vi "Get MAV ID.vi"(8 "Error In":errorcluster, 11 "Aircraft Index":u8) -> (0 "Error Out":errorcluster, 3 "Aircraft ID":u8)   [LabVIEW 2014]
uses:
  Get Aircraft Information.vi
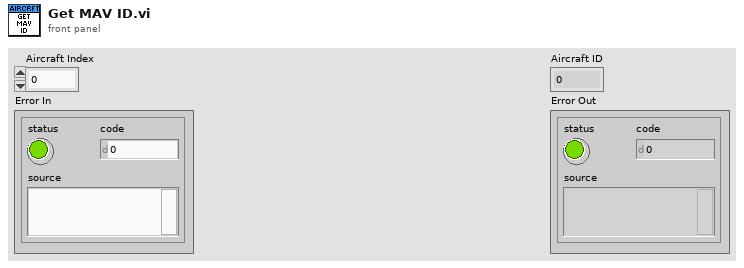
[diagram p1: front panel]
types:
  T1 = typedef "Drone Information.ctl" = cluster{"Aircraft ID":u8, "Tag ID":string, "System Status":string, "Base Mode":T2, "Armed/Disarmed":bool, "Battery Voltage":dbl, "Control Mode":T3, "Initialisation":u8, "Coms with aircraft good":bool, "Mode":string, "Mission Uploaded":bool}
  T2 = typedef "Base Mode.ctl" = cluster{"Custom Mode":bool, "Test Enabled":bool, "Autonomous Mode":bool, "Guided Mode":bool, "Stabilization Enabled":bool, "HIL Enabled":bool, "Manual Mode":bool, "Arm":bool}
  T3 = typedef "Aircraft Mode.ctl" = enum16{"Loiter", "Stabalise", "Failsafe", "Emergency Stop"}
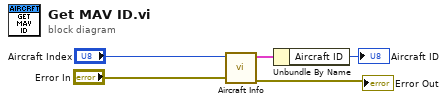
[diagram p0: block diagram]
diagram:
  n1 = call-poly "Aircraft Info.vi"("Error In"="Error In", "Aircraft ID"="Aircraft Index") -> ("Error Out"=→"Error Out":errorcluster, "Aircraft Information Out"=w4:T1)  [unwired: 8 in]
  n2 = Unbundle By Name(w4) -> ("Aircraft ID"=→"Aircraft ID":u8)
